vi "Generate_I2C.vi"(8 "Error_In":errorcluster, 10 "Mode":T1, 11 "7Bit_Address_In":refnum<class "7 Bit Address.lvclass">) -> (0 "Error_Out":errorcluster, 3 "7Bit_Address_Out":refnum<class "7 Bit Address.lvclass">)   [LabVIEW 2021, in "7 Bit Address.lvclass"]
doc: "Used to generate the I2C Waveform for 7 bit register"
uses:
  7 Bit Address.lvclass
  Controls/I2C_States.ctl
  Controls/Mode.ctl
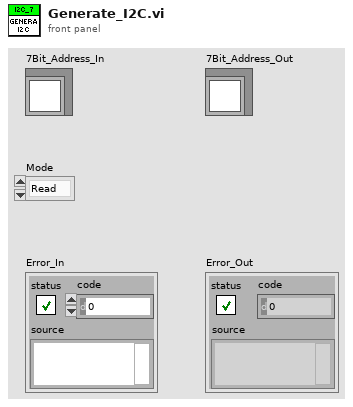
[diagram p1: front panel]
types:
  T1 = typedef "Mode.ctl" = enum16{"Read", "Write"}
  T2 = typedef "I2C_States.ctl" = enum16{"Start", "Byte", "Ack_Nack", "Stop"}
  T3 = typedef "I2C_Data.ctl" = cluster{"Vmin":dbl, "Vmax":dbl, "Input":string, "Off_Set (uS)":dbl, "T_HD_STA (uS)":dbl, "Sample_Per_Us":dbl, "T_HD_DAT (uS)":dbl, "T_SU_DAT (uS)":dbl, "Frequency (kHz)":dbl, "T_SU_STO":dbl, "T_Off (uS)":dbl, "T_On (uS)":dbl, "T_BUF":dbl, "Target_Address":u16, "Selected_Register_Address":u8, "Byte_Array":u8[], "Target_Name":string, "Register_Name":string[], "Register_Address":u8[], "Target_Type":T4, "Register_Data":string[]}
  T4 = typedef "Customized_Ring.ctl" = u16
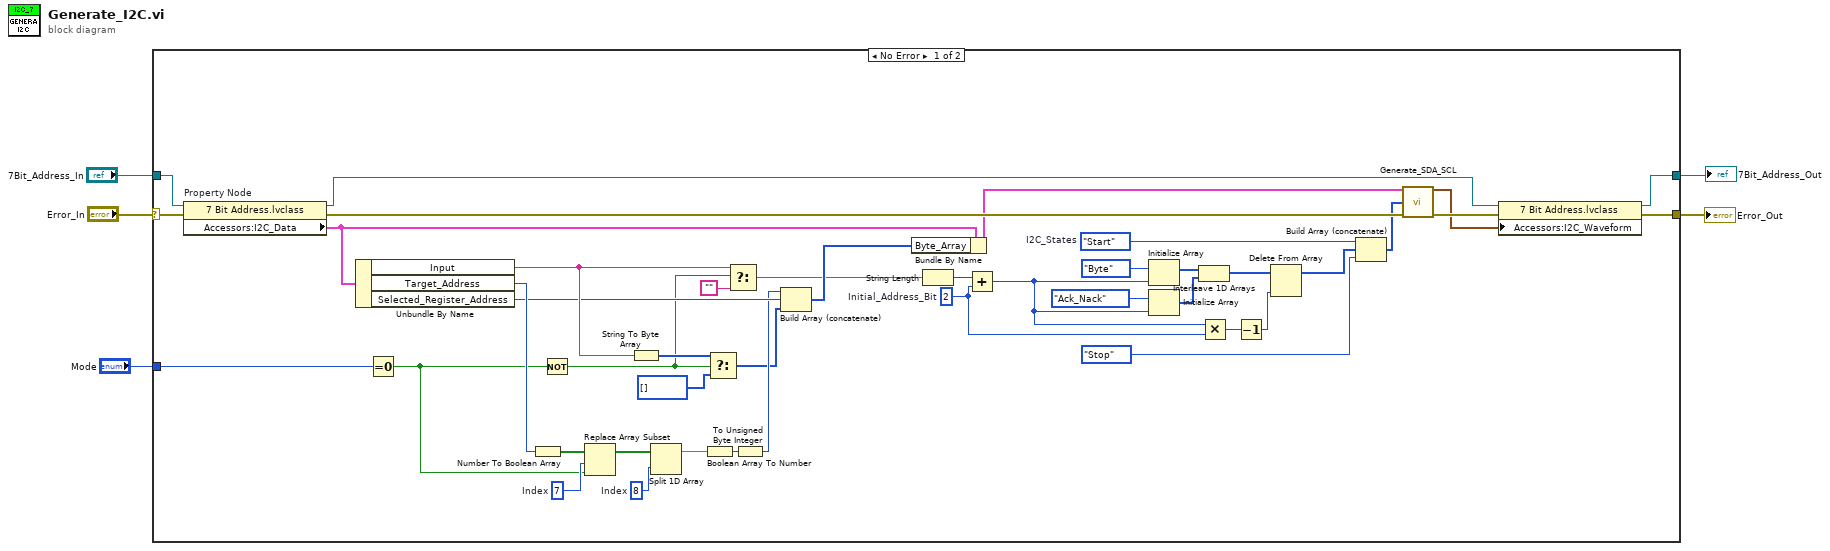
[diagram p0: block diagram]
diagram:
  n1 = case shown="No Error" "Error_In" {
    selector: "Error_In" -> [w47 w50]
    tunnel: [w26 w50] -> w5
    tunnel: [w27 w49] -> w4
    tunnel: "7Bit_Address_In" -> [w38 w49]
    tunnel: "Mode" -> [w34 _]
    frame No Error {
      w13 = 2  # Initial_Address_Bit
      w23 = 8  # Index
      w32 = 7  # Index
      w45 = I2C_States."Start"  # I2C_States
      n2 = property on="Property Node" class="7 Bit Address.lvclass"(reference=w38, error in=w47) -> (reference out=w37:refnum<class "7 Bit Address.lvclass">, error out=w46:errorcluster, "Accessors:I2C_Data"=w18:T3)
      n3 = Unbundle By Name(w18) -> ("Input"=w35:string, "Target_Address"=w31:u16, "Selected_Register_Address"=w29:u8)
      n4 = Equal To 0?(x=w34) -> (x = 0?=w19:bool)
      n5 = Number To Boolean Array(number=w31) -> (Boolean array=w33:bool[])
      n6 = Not(x=w19) -> (.not. x?=w7:bool)
      n7 = Replace Array Subset(array=w33, new element=w19, index=w32) -> (w25:bool[])
      n8 = String To Byte Array(string=w35) -> (unsigned byte array=w22:u8[])
      n9 = Split 1D Array(array=w25, index=w23) -> (first subarray=w24:bool[])  [unwired: 1 out]
      n10 = Boolean Array To Number(Boolean array=w24) -> (number=w30:u32)
      n11 = Select(t=w22, s=w7, f=u8[] []) -> (s? t:f=w21:u8[])
      n12 = Select(t=w35, s=w7, f="") -> (s? t:f=w8:string)
      n13 = To Unsigned Byte Integer(number=w30) -> (unsigned 8bit integer=w28:u8)
      n14 = Build Array (concatenate)(w28, w29, w21) -> (w16:u8[])
      n15 = Bundle By Name(cluster=w18, "Byte_Array"=w16) -> (w17:T3)
      n16 = String Length(string=w8) -> (length=w15:i32)
      n17 = Add(x=w15, y=w13) -> (x+y=w14:i32)
      n18 = Initialize Array(I2C_States."Byte" ("Enum"), w14) -> (w42:T2[])
      n19 = Initialize Array(I2C_States."Ack_Nack" ("element"), w14) -> (w41:T2[])
      n20 = Interleave 1D Arrays(w42, w41) -> (w11:T2[])
      n21 = Multiply(x=w14, y=w13) -> (x*y=w12:i32)
      n22 = Decrement(x=w12) -> (x-1=w9:i32)
      n23 = Delete From Array(array=w11, index=w9) -> (array with subset deleted=w10:T2[])  [unwired: 1 in, 1 out]
      n24 = Build Array (concatenate)(w45, w10, I2C_States."Stop" ("element")) -> (w39:T2[])
      n25 = call "Generate_SDA_SCL.vi"("Data"=w17, "Data_Sequence"=w39, "Error_In"=w46) -> ("Waveform Graph"=w36:waveform(dbl)[], "Error_Out"=w48:errorcluster)  [unwired: 11 in]
      n26 = property class="7 Bit Address.lvclass"(reference=w37, error in=w48, "Accessors:I2C_Waveform"=w36) -> (reference out=w27:refnum<class "7 Bit Address.lvclass">, error out=w26:errorcluster)
    }
    frame Error {
    }
  }
  "Error_Out" <- w5
  "7Bit_Address_Out" <- w4
